vi "chart combine.vi"(8 "error in (no error)":errorcluster, 10 "combined_chart":u32, 11 "chart":u32) -> (0 "error out":errorcluster)   [LabVIEW 8.6]
doc: "void chart_combine(lxw_chart chart, lxw_chart combined_chart);"
uses:
  pending_lvxlsxwriter/xlsxwriter.dll
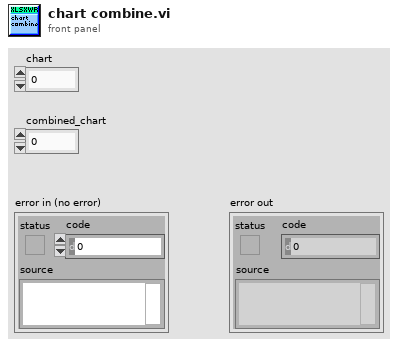
[diagram p1: front panel]
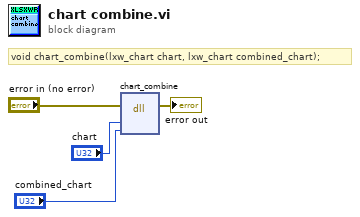
[diagram p0: block diagram]
diagram:
  # "void chart_combine(lxw_chart chart, lxw_chart combined_chart);"
  n1 = dll-call lib="C:/Users/WDAGUtilityAccount/Desktop/pending_lvxlsxwriter/xlsxwriter.*" fn="chart_combine"(error in="error in (no error)", "chart"="chart", "combined_chart"="combined_chart") -> (error out=→"error out":errorcluster)  [unwired: 5 in, 1 out]
